vi "HowToChangeRegimeTest.vi"() -> (3 "Were there any errors at all?":bool)   [LabVIEW 2013]
uses:
  Data/TypeDefs/Sailing Regimes.ctl
panel:
  in  "Boat speeds":dbl[](array[numeric])=[1.0, 0.0, 1.0, 1.0, 1.0, 0.1, 0.1]
  in  "Current regime inputs":T1[](array[typedef])=[enum."Upwind - Port Tack", enum."Upwind - Starboard Tack", enum."Reach - Port Tack", enum."Reach - Starboard Tack", enum."Reach - Port Tack", enum."Run - Port Tack", enum."Upwind - Starboard Tack", enum."Upwind - Port Tack"]
  in  "Desired regime inputs":T1[](array[typedef])=[enum."Upwind - Starboard Tack", enum."Upwind - Port Tack", enum."Run - Starboard Tack", enum."Reach - Port Tack", enum."Upwind - Starboard Tack", enum."Run - Starboard Tack", enum."Reach - Port Tack"]
  in  "Expected regime outputs":T1[](array[typedef])=[enum."Tack - Bow across wind", enum."Turn between Upwind/Reach - Starboard Tack", enum."Turn between Reach/Run - Port Tack", enum."Turn between Reach/Run - Starboard Tack", enum."Turn between Upwind/Reach - Port Tack", enum."Jibe - Stern across wind", enum."Turn between Upwind/Reach - Starboard Tack", enum."Upwind - Starboard Tack"]
  out "Actual regime outputs":T1[](array[typedef])=[enum."Tack - Bow across wind", enum."Turn between Upwind/Reach - Starboard Tack", enum."Turn between Reach/Run - Port Tack", enum."Turn between Reach/Run - Starboard Tack", enum."Turn between Upwind/Reach - Port Tack", enum."Jibe - Stern across wind", enum."Turn between Upwind/Reach - Starboard Tack"]
  out "Are chosen regimes right?":bool[](array[boolean])=[TRUE, TRUE, TRUE, TRUE, TRUE, TRUE, TRUE]
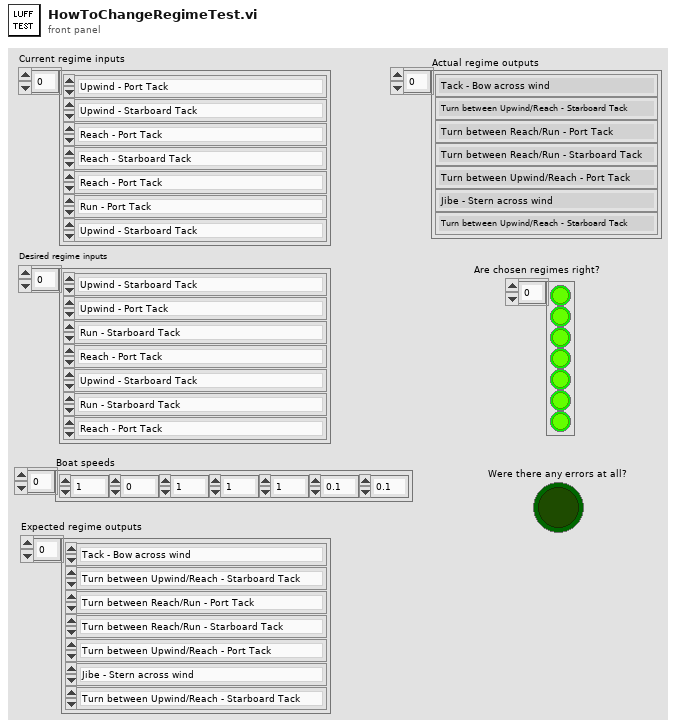
[diagram p1: front panel]
types:
  T1 = typedef "Sailing Regimes.ctl" = enum16{"Tack - Bow across wind", "Upwind - Starboard Tack", "Turn between Upwind/Reach - Starboard Tack", "Reach - Starboard Tack", "Turn between Reach/Run - Starboard Tack", "Run - Starboard Tack", "Jibe - Stern across wind", "Run - Port Tack", "Turn between Reach/Run - Port Tack", "Reach - Port Tack", "Turn between Upwind/Reach - Port Tack", "Upwind - Port Tack"}
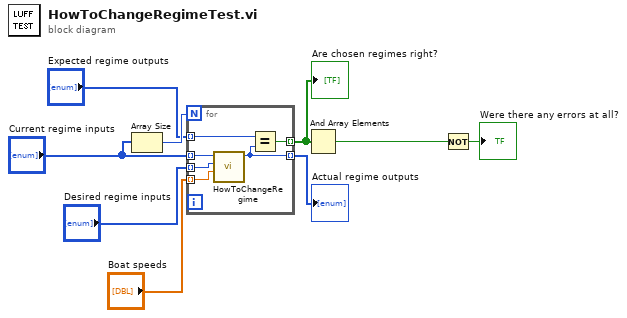
[diagram p0: block diagram]
diagram:
  n1 = Array Size(array="Current regime inputs") -> (size(s)=w9:i32)
  n2 = for {
    N: w9 -> [_]
    tunnel: "Expected regime outputs" -> [w15] mode=indexing
    tunnel: [w14] -> w8 mode=indexing
    tunnel: "Current regime inputs" -> [w12] mode=indexing
    tunnel: [w13] -> w4 mode=indexing
    tunnel: "Desired regime inputs" -> [w11] mode=indexing
    tunnel: "Boat speeds" -> [w10] mode=indexing
    n3 = call "HowToChangeRegime.vi"("Boat speed (m/s)"=w10, "Desired Sailing Regime"=w11, "Current Sailing Regime"=w12) -> ("Output sailing regime"=w13:T1)  [unwired: 8 in]
    n4 = Equal?(x=w15, y=w13) -> (x = y?=w14:bool)
  }
  "Are chosen regimes right?" <- w8
  "Actual regime outputs" <- w4
  n5 = And Array Elements(Boolean array=w8) -> (logical AND=w6:bool)
  n6 = Not(x=w6) -> (.not. x?=→"Were there any errors at all?":bool)
